vi "Byte_Array_To_12_Bit_Array.vi"(1 "Byte-Array":u8[](array[numeric])) -> (0 "12-Bit-Array":u16[](array[numeric]))   [LabVIEW 2010]
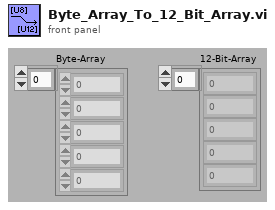
[diagram p1: front panel]
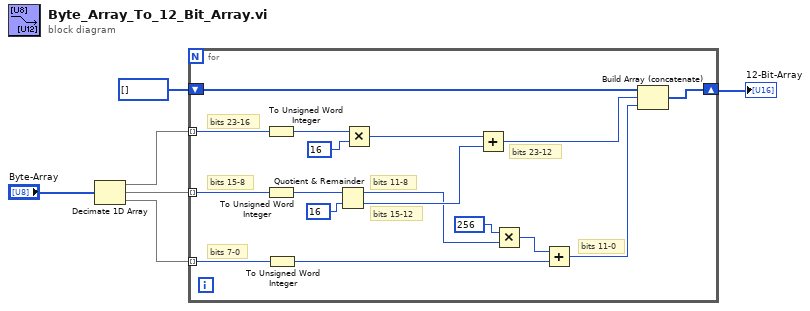
[diagram p0: block diagram]
diagram:
  n1 = Decimate 1D Array("Byte-Array") -> (w6:u8[], w5:u8[], w4:u8[])
  n2 = for {
    tunnel: w6 -> [w9] mode=indexing
    tunnel: w5 -> [w12] mode=indexing
    tunnel: w4 -> [w13] mode=indexing
    shift-right: [w16] -> w1
    shift-left: u16[] [] -> [w17]
    # "bits 11-0"
    # "bits 11-8"
    # "bits 15-12"
    # "bits 23-12"
    # "bits 7-0"
    # "bits 15-8"
    # "bits 23-16"
    n3 = To Unsigned Word Integer(number=w9) -> (unsigned 16bit integer=w10:u16)
    n4 = To Unsigned Word Integer(number=w12) -> (unsigned 16bit integer=w11:u16)
    n5 = To Unsigned Word Integer(number=w13) -> (unsigned 16bit integer=w14:u16)
    n6 = Quotient & Remainder(x=w11, y=u16 16) -> (x-y*floor(x/y)=w7:u16, floor(x/y)=w18:u16)
    n7 = Multiply(x=w10, y=u16 16) -> (x*y=w22:u16)
    n8 = Add(x=w22, y=w18) -> (x+y=w21:u16)
    n9 = Multiply(x=u16 256, y=w7) -> (x*y=w15:u16)
    n10 = Add(x=w15, y=w14) -> (x+y=w20:u16)
    n11 = Build Array (concatenate)(w17, w21, w20) -> (w16:u16[])
  }
  "12-Bit-Array" <- w1
